vi "incrementmotor.vi"() -> ()   [LabVIEW 2014]
panel:
  out "Position Out":i32
  in  "Current Position":i32
  in  "Desired Position":i32
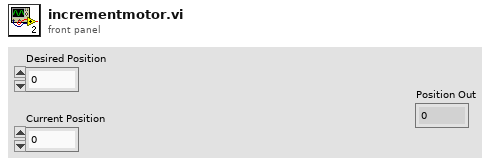
[diagram p1: front panel]
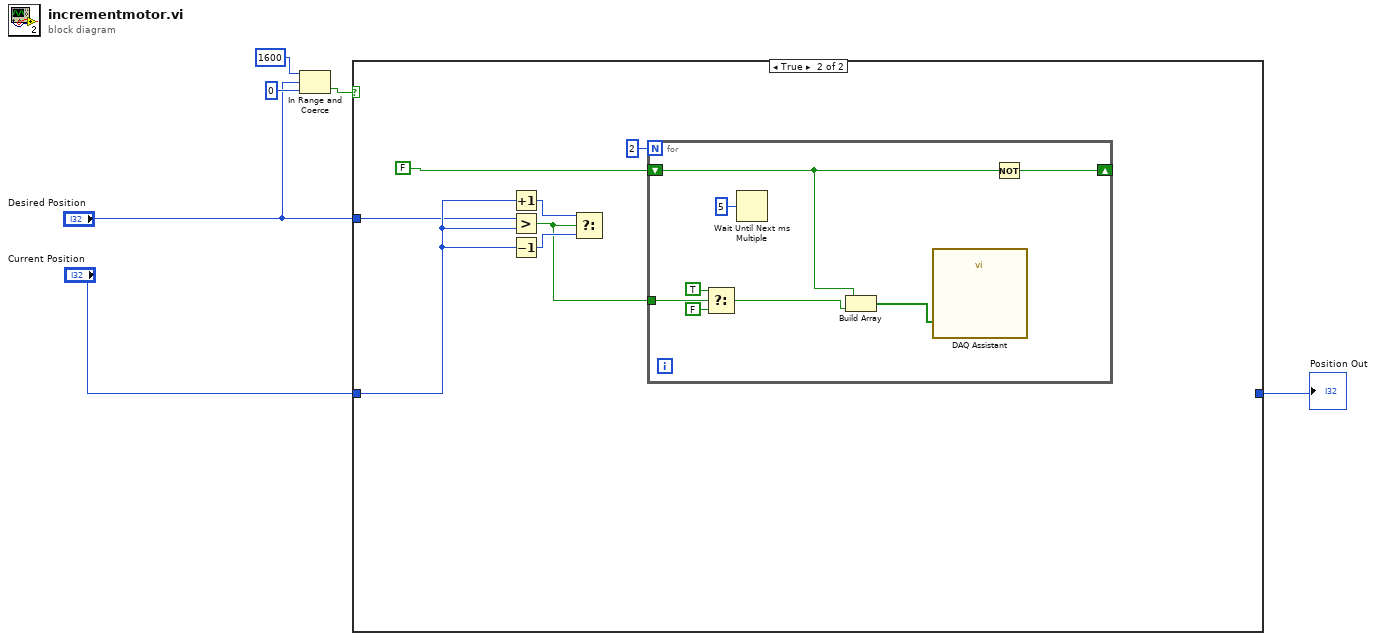
[diagram p0: block diagram]
diagram:
  n1 = In Range and Coerce(upper limit=1600, x="Desired Position", lower limit=0) -> (In Range?=w5:bool)  [unwired: 1 out]
  n2 = case shown="True" w5 {
    tunnel: [w7 _] -> w6
    tunnel: "Current Position" -> [w7 w13]
    tunnel: "Desired Position" -> [_ w12]
    frame False {
    }
    frame True {
      n3 = Increment(x=w13) -> (x+1=w11:i32)
      n4 = Greater?(x=w12, y=w13) -> (0:w9:bool)
      n5 = Decrement(x=w13) -> (x-1=w10:i32)
      n6 = Select(t=w11, s=w9, f=w10) -> ()  [unwired: 1 out]
      n7 = for {
        N: 2 -> [_]
        tunnel: w9 -> [w18]
        shift-right: [w15] -> _
        shift-left: FALSE -> [w22]
        n8 = Select(t=TRUE, s=w18, f=FALSE) -> (s? t:f=w21:bool)
        n9 = Wait Until Next ms Multiple(millisecond multiple=u32 5) -> ()  [unwired: 1 out]
        n10 = Build Array(w22, w21) -> (w16:bool[])
        n11 = call "DAQ Assistant"("data"=w16) -> ()  [unwired: 17 in, 2 out]
        n12 = Not(x=w22) -> (.not. x?=w15:bool)
      }
    }
  }
  "Position Out" <- w6
